vi "FTW-TransferClient-Callback-StatusUpload.vi"(4 "Initial Parameters":T1 {"Initial Time" format="%.4psec"}, 5 "Event Data":cluster{"sender":refnum<k24>, "e":refnum<k24>}, 6 "Control Ref":refnum<k24>, 7 "Event Common Data":T2) -> ()   [LabVIEW 2015]
uses:
  FTW-TransferClient-TransferStatus.ctl
panel:
  # "Inputs"
  # "Outputs"
  # "No Outputs - this VI\nis fire and forget"
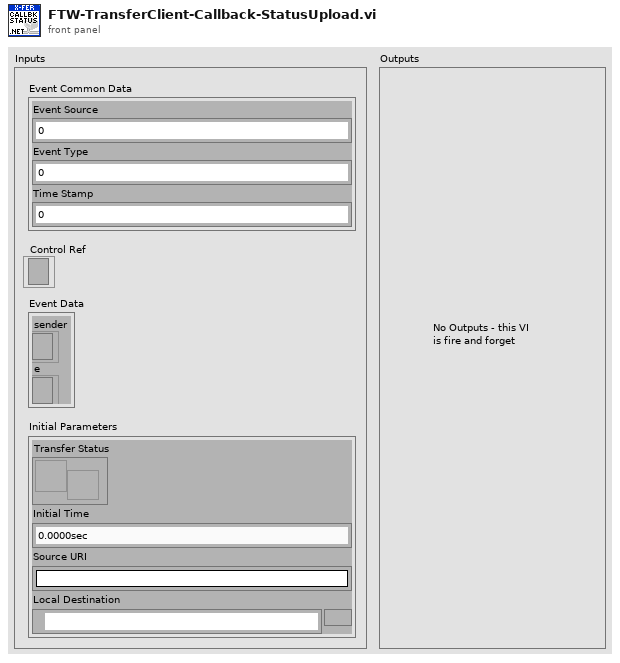
[diagram p1: front panel]
types:
  T1 = cluster{"Transfer Status":refnum<user-event>, "Initial Time":dbl, "Source URI":string, "Local Destination":path}
  T2 = cluster{"Event Source":i32, "Event Type":u32, "Time Stamp":u32}
  T3 = typedef "FTW-TransferClient-TransferStatus.ctl" = cluster{"Remote URI":string, "Local Filepath":path, "Cancelled?":bool, "Error?":bool, "Error Message":string, "Elapsed Time":dbl}
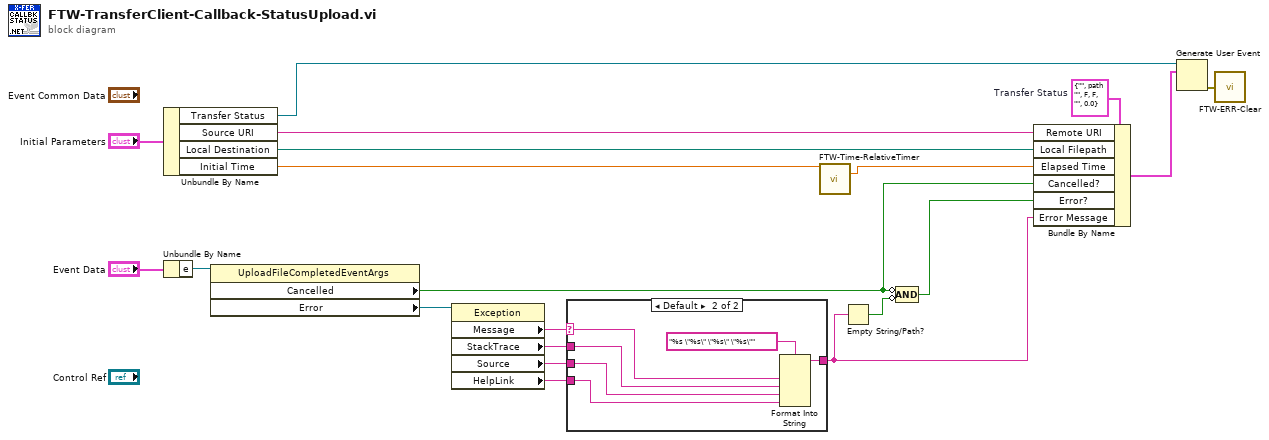
[diagram p0: block diagram]
diagram:
  w9 = T3 {"Remote URI"="", "Local Filepath"=path "", "Cancelled?"=FALSE, "Error?"=FALSE, "Error Message"="", "Elapsed Time"=0.0}  # Transfer Status
  n1 = Unbundle By Name("Initial Parameters") -> ("Transfer Status"=w3:refnum<user-event>, "Source URI"=w8:string, "Local Destination"=w7:path, "Initial Time"=w2:dbl)
  n2 = Unbundle By Name("Event Data") -> ("e"=w18:refnum<k24>)
  n3 = property class="UploadFileCompletedEventArgs"(reference=w18) -> ("Cancelled"=w6:bool, "Error"=w16:refnum<k24>)  [unwired: 1 in, 2 out]
  n4 = property class="Exception"(reference=w16) -> ("Message"=w14:string, "StackTrace"=w15:string, "Source"=w13:string, "HelpLink"=w12:string)  [unwired: 1 in, 2 out]
  n5 = case shown="Default" w14 {
    selector: w14 -> [_ w24]
    tunnel: w15 -> [_ w23]
    tunnel: [_ w25] -> w4
    tunnel: w13 -> [_ w22]
    tunnel: w12 -> [_ w21]
    frame "" {
    }
    frame Default {
      n6 = Format Into String(format string="%s \"%s\" \"%s\" \"%s\"", w24, w23, w22, w21) -> (resulting string=w25:string)  [unwired: 2 in, 1 out]
    }
  }
  n7 = call "FTW-Time-RelativeTimer.vi"("Previous Timer Value"=w2) -> ("Elapsed Time"=w1:dbl)  [unwired: 12 in, 2 out]
  n8 = Empty String/Path?(string/path=w4) -> (empty?=w17:bool)
  n9 = Compound Arithmetic op=AND(invert w6, invert w17) -> (w5:bool)
  n10 = Bundle By Name(cluster=w9, "Remote URI"=w8, "Local Filepath"=w7, "Elapsed Time"=w1, "Cancelled?"=w6, "Error?"=w5, "Error Message"=w4) -> (w11:T3)
  n11 = Generate User Event(user event=w3, event data cluster=w11) -> (error out=w10:errorcluster)  [unwired: 2 in, 1 out]
  n12 = call "FTW-ERR-Clear.vi"("error to snuff"=w10) -> ()  [unwired: 1 out]
